vi "Meas Result Update View.vi"(8 "error in":errorcluster, 10 "gui refs":T29, 11 "meas":T3={"swp cfg"={"N"=0, "R"=0, "f list"=[], "smpl delay"=0.0, "set delay"=0.0, "set delay np"=0.0, "meas root"=path "", "meas name"="", "meas a-index"=FALSE, "rnd sweep"=FALSE, "mode"=enum."Frequency", "swp mode"=enum."Linear", "avg"=0, "subrec"=0, "multi-freq"=FALSE, "selfcal"=FALSE, "selfcal period [h]"=0.0}, "bridge"={"type"=enum."TWM client", "TWM"={"pipe name"="", "parameters"=[], "handle"=0, "fixed aper [s]"=0.0, "f-list [Hz]"=[], "discrete f-list"=FALSE, "unc mode"=enum."None", "unc mcc"=0, "unc first"=FALSE, "alg id"=enum."TWM-LowZ - Low Z measurement"}, "last f"=0.0, "bias comp"={"bias type"=enum."dummy", "VISA"="", "Enable"=FALSE, "channel qu"=[], "channel Uinit"=[]}, "sim mode"=enum."Generic RLC network", "channel idns"=[], "sim phases"=1}, "src"={"type"=enum."Tektronix AFG3101C", "afg"={"VISA"="", "const"=0.0, "gen DC"=FALSE, "ext ref"=FALSE}, "cDAQ dds"={"device"="", "channels"=[], "mclk source"="", "mclk [Hz]"=0.0, "fs [Hz]"=0.0, "block [s]"=0.0, "buf [s]"=0.0, "task"="", "cmd queue"=refnum, "proc ref"=refnum, "smpl clock out"="/cDAQ3/PFI0", "export smpl clock"=FALSE, "DC ofs [V]"=[], "timebase source"="", "timebase mode"=enum."Local", "dither"=enum."Disabled", "dither level"=0.0, "phase [rad]"=[]}, "gain [V/A]"=1.0, "F5xxx session"={"VISA"="", "mode"=enum."AC voltage", "Earth on"=FALSE, "Ext ref lock"=FALSE}}, "results"=refnum, "dvm"={"type"=enum."Disabled", "F5790"={"VISA"="", "Input"=enum."input 1", "Digital filter restart"=enum."medium", "hi resolution"=enum."off", "Digital filter mode"=enum."off", "ext guard"=FALSE}}} {"src"."cDAQ dds"."channels" min=0 step=1; "bridge"."TWM"."f-list [Hz]" format="%#_6p"; "swp cfg"."f list"."bias" format="%#_3p"; "swp cfg"."f list"."level" format="%#_3p"; "swp cfg"."f list"."fs [Hz]" format="%#_5p"; "swp cfg"."f list"."time [s]" format="%#_3p"; "swp cfg"."f list"."f/fs" format="%#_3p"; "swp cfg"."f list"."periods" format="%#_3f"; "swp cfg"."f list"."f [Hz]" format="%#_5p"}) -> (0 "error out":errorcluster, 3 "was modified?":bool)   [LabVIEW 2020]
doc: "Update results view."
uses:
  Meas Result GUI References.ctl
  Meas Result Freq Format.ctl
  Meas Results Sweep Data Uncertainty Mode.ctl
  Meas Result 4TP Impedance Mode.ctl
  Impedance Equivalent Circuit.ctl
  meas session.ctl
  Meas Sweep Config.ctl
  Meas Freq Info.ctl
  meas_swp_mode.ctl
  meas_sweep_flist_mode.ctl
  bridge/Bridge Session.ctl
  bridge/Bridge Type.ctl
  drivers/TWM client/TWM Session.ctl
  drivers/TWM client/TWM parameters.ctl
  drivers/TWM client/Meas Proc QWTB Uncertainty Mode.ctl
  bridge/Bridge Algorithm.ctl
  bridge/Bridge Bias Session.ctl
  bridge/Bridge Bias Type.ctl
  bridge/Bridge Sim Mode.ctl
  source/Source Session.ctl
  source/Source Type.ctl
  drivers/AFG3101C/AFG3101C Session.ctl
  drivers/cDAQ DDS/cDAQ DDS Session.ctl
  drivers/cDAQ DDS/cDAQ DDS Setup.ctl
  drivers/cDAQ DDS/cDAQ DDS Timebase Mode.ctl
  drivers/cDAQ DDS/cDAQ DDS Dither.ctl
  drivers/Fluke 5XXX/top_lev/F5xxx_session.ctl
  drivers/Fluke 5XXX/top_lev/F5xxx_output_mode.ctl
  Meas Results Ref.ctl
  Meas Results.ctl
  bridge/Bridge Frequency Readings Data.ctl
  drivers/TWM client/Meas Proc QWTB Spectrum Data.ctl
  drivers/TWM client/TWM Phase Info.ctl
  dvm/dvm session.ctl
  dvm/dvm type.ctl
  drivers/Fluke 5790A/top_level/F5790 session.ctl
  Meas Result Major Format.ctl
  Meas Result Deviation Format.ctl
  varilib/varilib.lvlib
panel:
  in  "mjr dev fmt":T1 caption="Enum"
  in  "mjr fmt":T2=enum."%_5p"
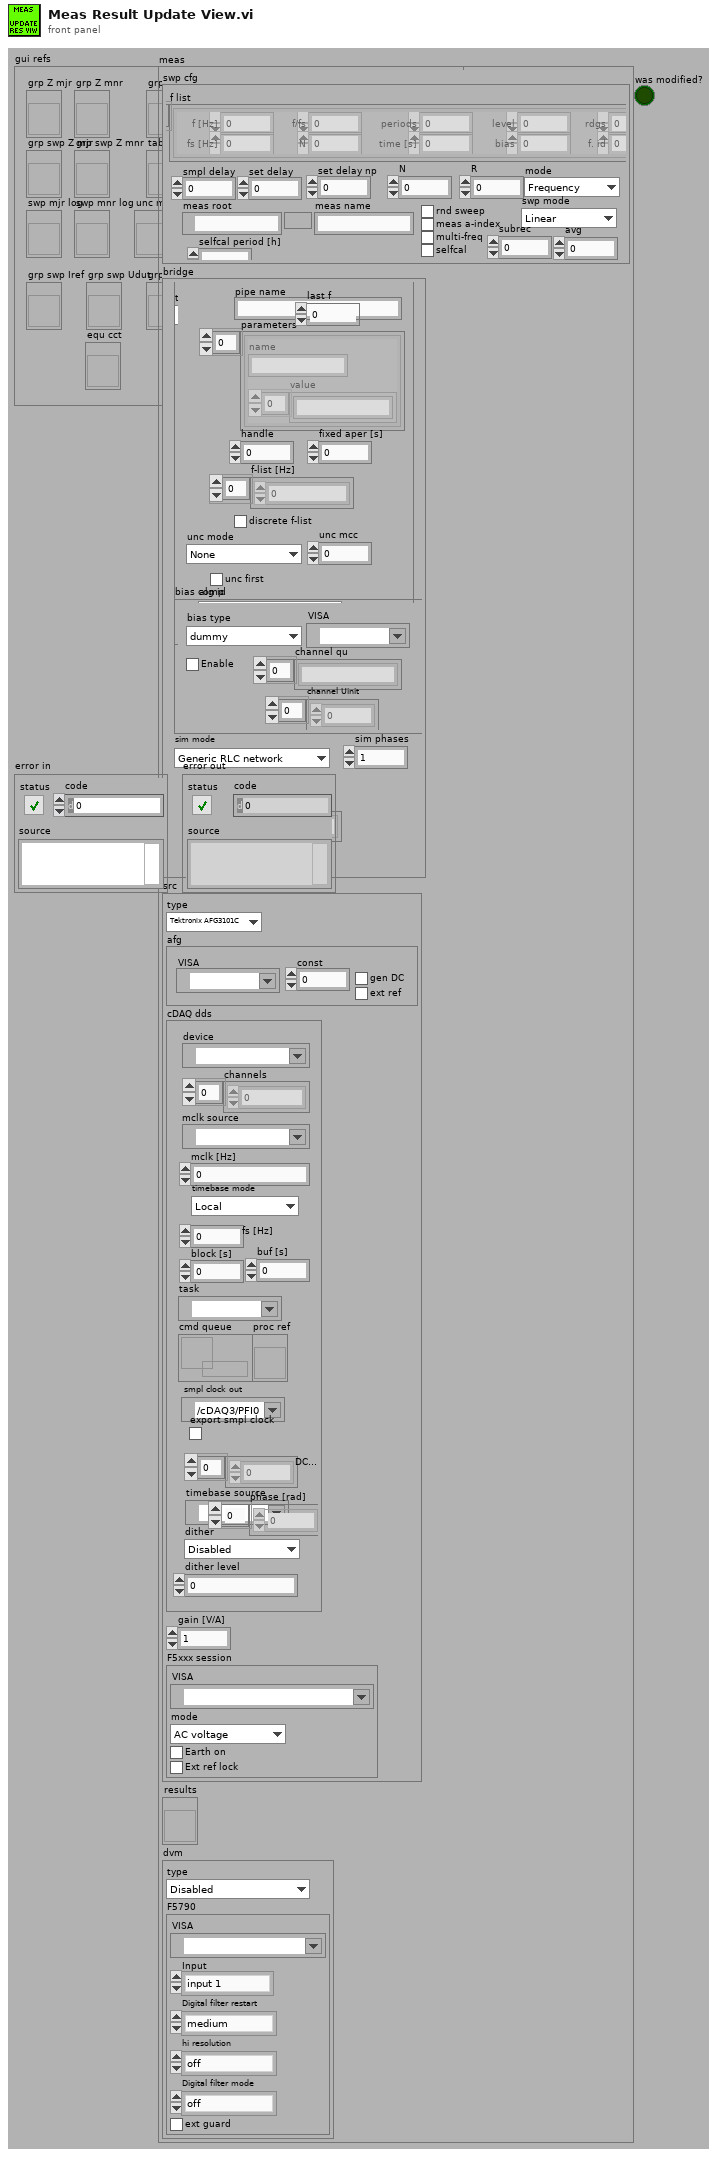
[diagram p1: front panel]
types:
  T1 = typedef "Meas Result Deviation Format.ctl" = enum16{"dev(abs)", "dev(%)", "dev(ppm)", "u(abs)", "u(%)", "u(ppm)"}
  T2 = typedef "Meas Result Major Format.ctl" = enum16{"%_3p", "%_4p", "%_5p", "%_6p", "%_7p", "%_8p", "%_5f", "%_6f", "%_7f", "%_8f", "%_5e", "%_6e", "%_7e", "%_8e", "%.4f", "%.5f", "%.6f", "%.7f"}
  T3 = typedef "meas session.ctl" = cluster{"swp cfg":T4, "bridge":T8, "src":T17, "results":T25, "dvm":T26}
  T4 = typedef "Meas Sweep Config.ctl" = cluster{"N":i32, "R":i32, "f list":T5[], "smpl delay":dbl, "set delay":dbl, "set delay np":dbl, "meas root":path, "meas name":string, "meas a-index":bool, "rnd sweep":bool, "mode":T6, "swp mode":T7, "avg":i32, "subrec":i32, "multi-freq":bool, "selfcal":bool, "selfcal period [h]":dbl}
  T5 = typedef "Meas Freq Info.ctl" = cluster{"f [Hz]":dbl, "periods":dbl, "f/fs":dbl, "time [s]":dbl, "fs [Hz]":dbl, "N":i32, "level":dbl, "bias":dbl, "rdgs":i32, "f. id":i32}
  T6 = typedef "meas_swp_mode.ctl" = enum16{"Frequency", "Level", "Bias"}
  T7 = typedef "meas_sweep_flist_mode.ctl" = enum16{"Linear", "Log10"}
  T8 = typedef "Bridge Session.ctl" = cluster{"type":T9, "TWM":T10, "last f":dbl, "bias comp":T14, "sim mode":T16, "channel idns":string[], "sim phases":i32}
  T9 = typedef "Bridge Type.ctl" = enum16{"TWM client", "dummy"}
  T10 = typedef "TWM Session.ctl" = cluster{"pipe name":string, "parameters":T11[], "handle":i32, "fixed aper [s]":dbl, "f-list [Hz]":dbl[], "discrete f-list":bool, "unc mode":T12, "unc mcc":i32, "unc first":bool, "alg id":T13}
  T11 = typedef "TWM parameters.ctl" = cluster{"name":string, "value":string[]}
  T12 = typedef "Meas Proc QWTB Uncertainty Mode.ctl" = enum16{"None", "GUF", "Monte Carlo"}
  T13 = typedef "Bridge Algorithm.ctl" = enum16{"TWM-LowZ - Low Z measurement", "TWM-InpZ - Digitizer input Z measurement", "TWM-TIAZ - High Z using TIA"}
  T14 = typedef "Bridge Bias Session.ctl" = cluster{"bias type":T15, "VISA":refnum<visa-resource-name>, "Enable":bool, "channel qu":string[], "channel Uinit":dbl[]}
  T15 = typedef "Bridge Bias Type.ctl" = enum16{"dummy", "CMI LiBbias V1.0"}
  T16 = typedef "Bridge Sim Mode.ctl" = enum16{"Generic RLC network", "Interchannel transfer", "Input impedance"}
  T17 = typedef "Source Session.ctl" = cluster{"type":T18, "afg":T19, "cDAQ dds":T20, "gain [V/A]":dbl, "F5xxx session":T23}
  T18 = typedef "Source Type.ctl" = enum16{"Tektronix AFG3101C", "cDAQ DAC", "Fluke 5xxx", "Agilent 33120A", "dummy"}
  T19 = typedef "AFG3101C Session.ctl" = cluster{"VISA":refnum<visa-resource-name>, "const":dbl, "gen DC":bool, "ext ref":bool}
  T20 = typedef "cDAQ DDS Session.ctl" = cluster{"device":tag, "channels":i32[], "mclk source":tag, "mclk [Hz]":dbl, "fs [Hz]":dbl, "block [s]":dbl, "buf [s]":dbl, "task":refnum<k21>, "cmd queue":refnum<queue>, "proc ref":refnum<vi>, "smpl clock out":tag, "export smpl clock":bool, "DC ofs [V]":dbl[], "timebase source":tag, "timebase mode":T21, "dither":T22, "dither level":dbl, "phase [rad]":dbl[]}
  T21 = typedef "cDAQ DDS Timebase Mode.ctl" = enum16{"Local", "Take from ADC (e.g. NI 9238)", "Other source"}
  T22 = typedef "cDAQ DDS Dither.ctl" = enum16{"Disabled", "Gaussian"}
  T23 = typedef "F5xxx_session.ctl" = cluster{"VISA":refnum<visa-resource-name>, "mode":T24, "Earth on":bool, "Ext ref lock":bool}
  T24 = typedef "F5xxx_output_mode.ctl" = enum16{"AC voltage", "AC current"}
  T25 = typedef "Meas Results Ref.ctl" = refnum<vi>
  T26 = typedef "dvm session.ctl" = cluster{"type":T27, "F5790":T28}
  T27 = typedef "dvm type.ctl" = enum16{"Disabled", "Simulated", "Fluke 5790A"}
  T28 = typedef "F5790 session.ctl" = cluster{"VISA":refnum<visa-resource-name>, "Input":enum16{"input 1", "input 2", "wide-band"}, "Digital filter restart":enum16{"medium", "fine", "coarse"}, "hi resolution":enum16{"off", "on"}, "Digital filter mode":enum16{"off", "fast", "medium", "slow"}, "ext guard":bool}
  T29 = typedef "Meas Result GUI References.ctl" = cluster{"grp Z mjr":refnum<vi>, "grp Z mnr":refnum<vi>, "grp swp Z mjr":refnum<vi>, "grp swp Z mnr":refnum<vi>, "swp mjr log":refnum<vi>, "swp mnr log":refnum<vi>, "grp ref":refnum<vi>, "tab swp":refnum<vi>, "mjr fmt":refnum<vi>, "mnr fmt":refnum<vi>, "mjr dev fmt":refnum<vi>, "mnr dev fmt":refnum<vi>, "res frq fmt":refnum<vi>, "unc mode":refnum<vi>, "mode 4TP":refnum<vi>, "grp spec 0":refnum<vi>, "grp spec 1":refnum<vi>, "cb spec log":refnum<vi>, "res pid":refnum<vi>, "res fid":refnum<vi>, "grp swp cplx":refnum<vi>, "cb grp inv Xs":refnum<vi>, "grp swp Iref":refnum<vi>, "grp swp Udut":refnum<vi>, "grp swp Udvm":refnum<vi>, "swp Iref log":refnum<vi>, "swp Udut log":refnum<vi>, "swp Udvm log":refnum<vi>, "grp ui ref":refnum<vi>, "grp Iref":refnum<vi>, "grp Udut":refnum<vi>, "grp Udvm":refnum<vi>, "equ cct":refnum<vi>}
  T30 = typedef "Meas Results.ctl" = cluster{"freqs":T31[][], "locked":bool, "last fid":i32, "modified":bool, "mjr name":string, "mnr name":string, "last spectra":T32[][], "saved?":bool, "TWM phase":T33[], "time start":timestamp, "time stop":timestamp, "equ cct":string}
  T31 = typedef "Bridge Frequency Readings Data.ctl" = cluster{"Udut":dbl[], "Iref":dbl[], "Udc":dbl[], "Idc":dbl[], "mjr":dbl[], "mnr":dbl[], "mjr_sh":dbl[], "mnr_sh":dbl[], "u(mjr)":dbl[], "u(mnr)":dbl[], "ua2(mjr)":dbl[], "ua2(mnr)":dbl[], "n":i32, "f [Hz]":dbl, "fs [Hz]":dbl, "aperture [s]":dbl, "Udvm":dbl[], "u(Udvm) [V]":dbl}
  T32 = typedef "Meas Proc QWTB Spectrum Data.ctl" = cluster{"x":sgl[], "y":sgl[], "label":string}
  T33 = typedef "TWM Phase Info.ctl" = cluster{"ref chn id (I)":string, "dut chn id (U)":string, "ref chn range [V]":dbl, "dut chn range [V]":dbl, "aperture [s]":dbl, "fs [Hz]":dbl, "ref chn transducer (I)":string, "dut chn transducer (U)":string}
  T34 = typedef "Impedance Equivalent Circuit.ctl" = enum16{"Keep original", "Rs-Xs", "Gp-Bp", "Z-phid", "Z-phir", "Y-phid", "Y-phir", "Cp-D", "Cp-Q", "Cp-Rp", "Cp-Gp", "Cs-D", "Cs-Q", "Cs-Rs", "Ls-Rs", "Ls-Q", "Rs-Tau"}
  T35 = typedef "Meas Result 4TP Impedance Mode.ctl" = enum16{"4T/4TP total Z", "4TP-shield Z"}
  T36 = typedef "Impedance Equivalent Circuit Type Info.ctl" = cluster{"major":string, "major unit":string, "minor":string, "minor unit":string, "combined":string, "major+unit":string, "minor+unit":string}
  T37 = typedef "Meas Results Sweep Data Uncertainty Mode.ctl" = enum16{"ua(y)", "ua(y) (p=95%)", "uc(y) (p=95%)"}
  T38 = typedef "Meas Quantity Names.ctl" = cluster{"mjr name":string, "mnr name":string, "mjr unit":string, "mnr unit":string, "mjr full":string, "mnr full":string}
  T39 = typedef "Meas Results Sweep Data.ctl" = cluster{"Udut":dbl[], "Iref":dbl[], "Udc":dbl[], "Idc":dbl[], "mjr":dbl[], "mnr":dbl[], "mjr_sh":dbl[], "mnr_sh":dbl[], "f [Hz]":dbl[], "n [-]":i32[], "fs [Hz]":dbl[], "aperture [s]":dbl[], "Udvm":dbl[]}
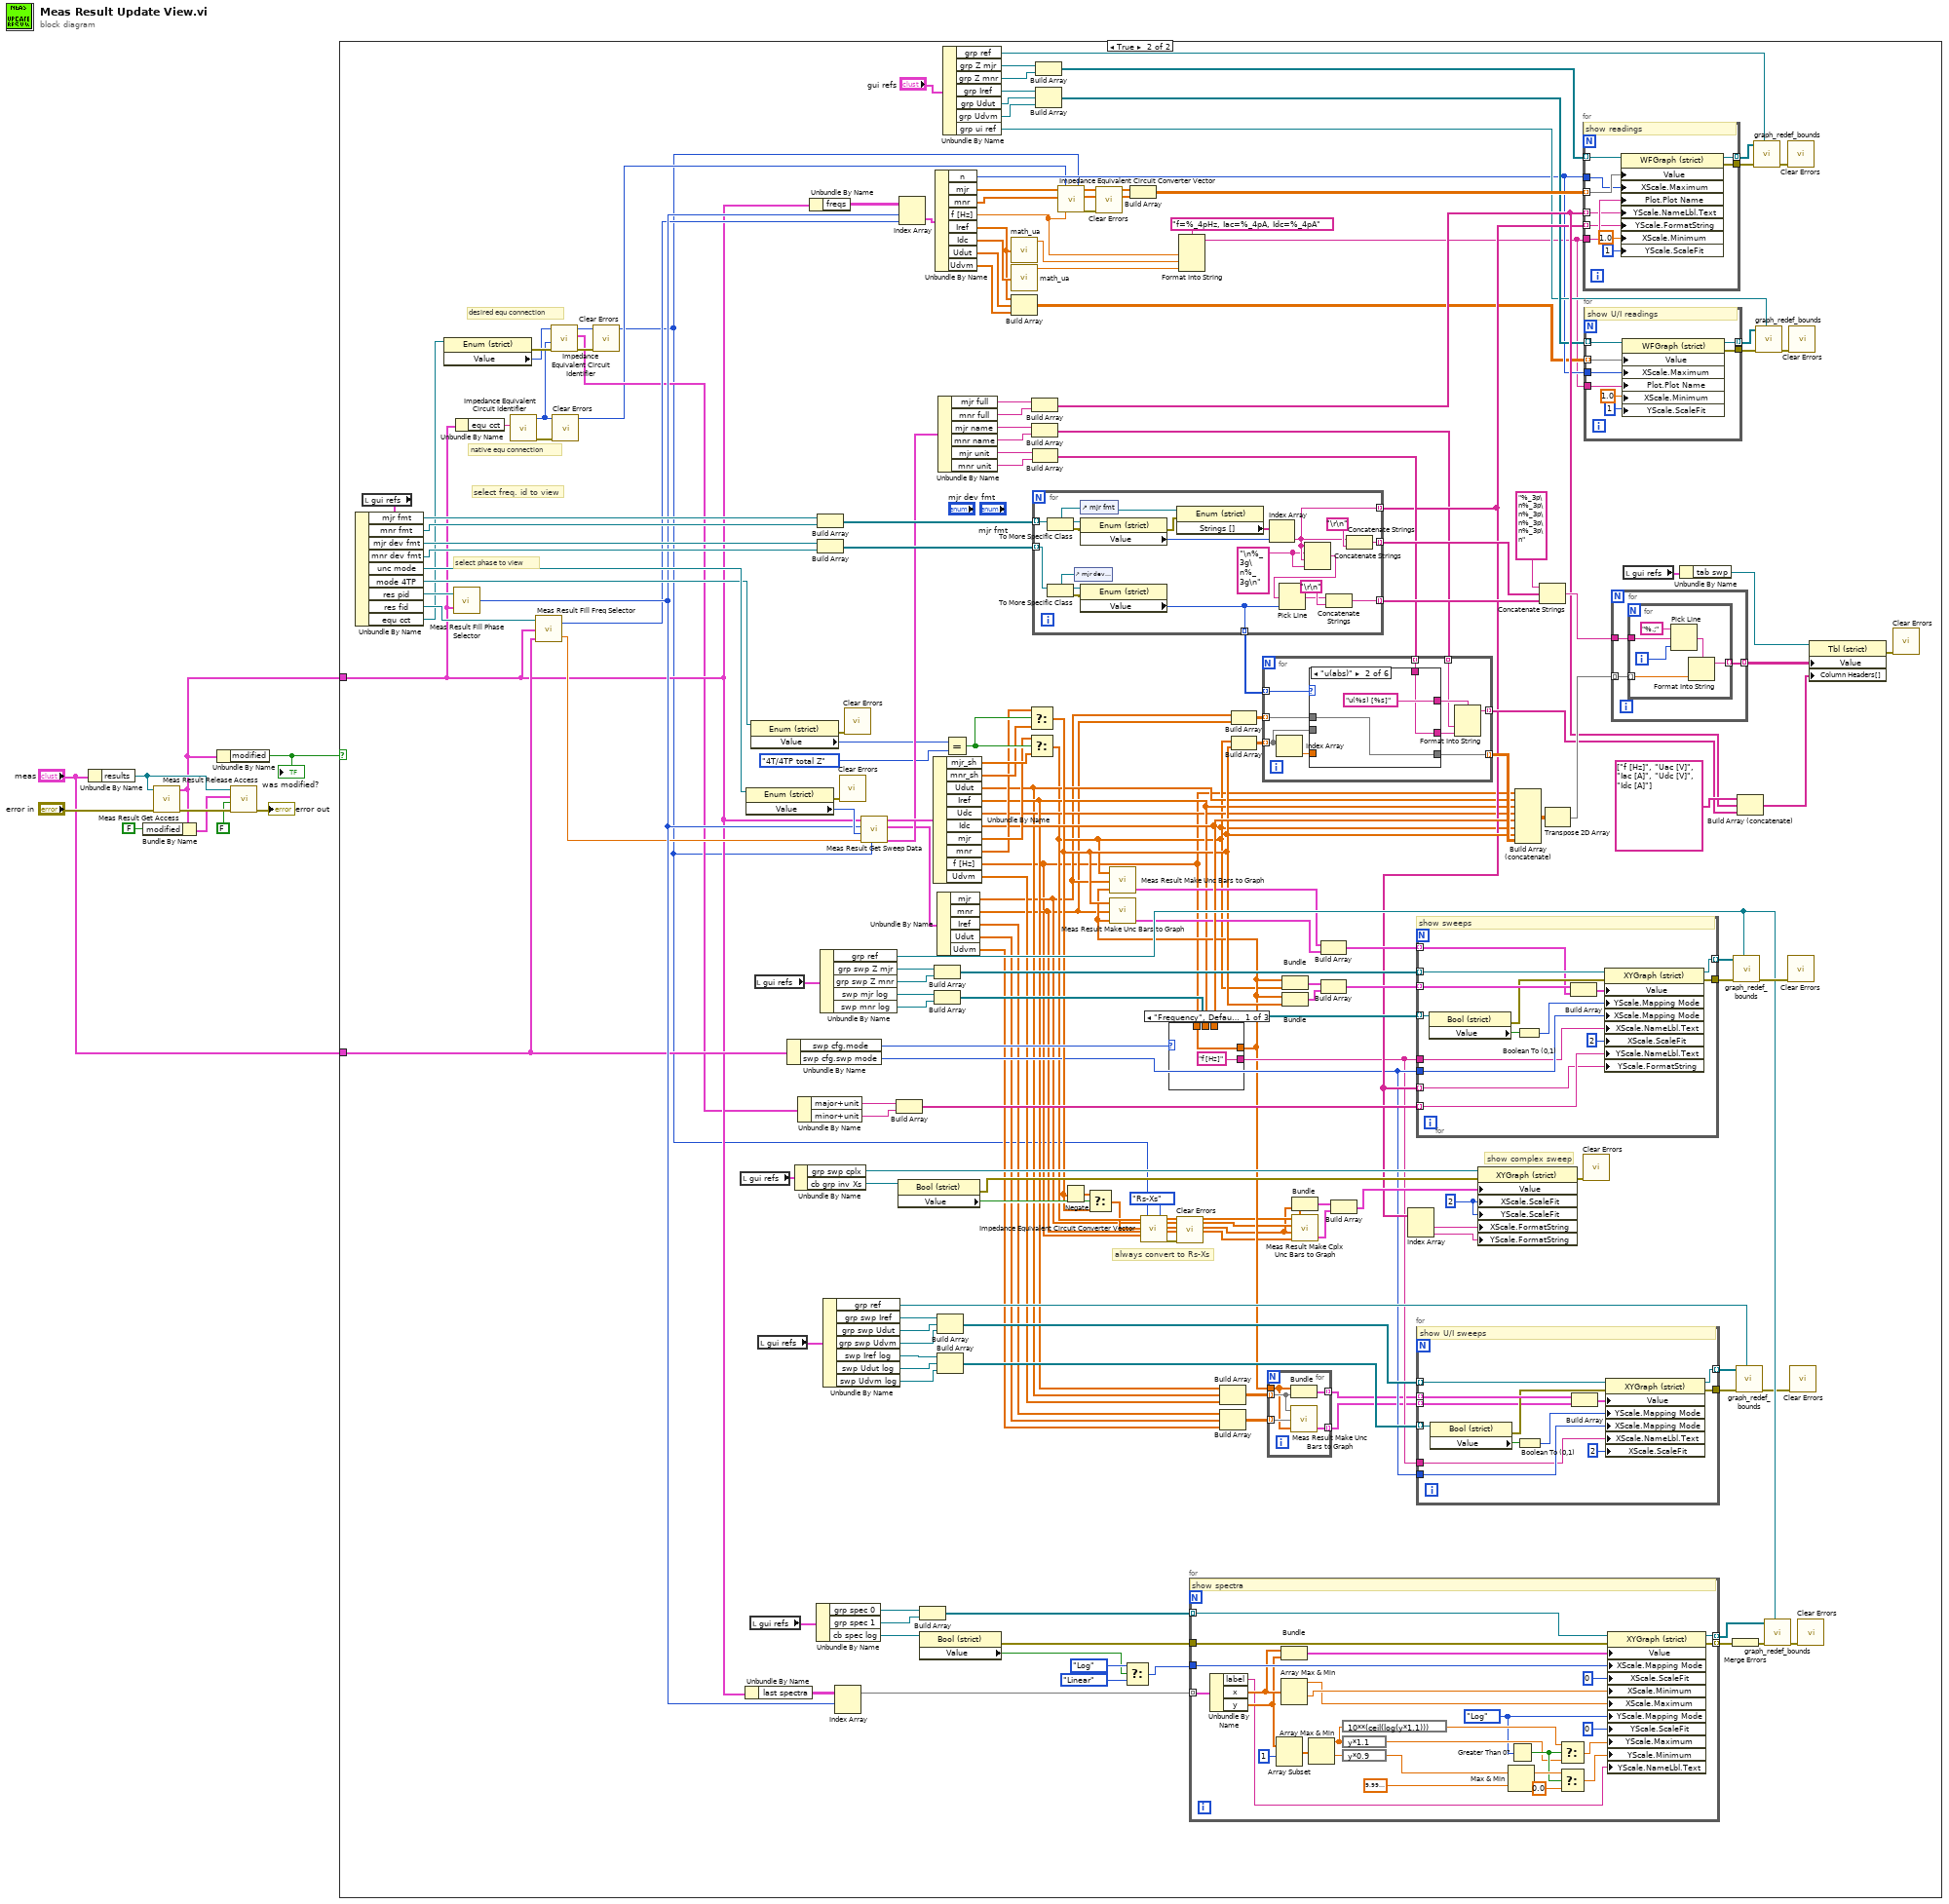
[diagram p0: block diagram]
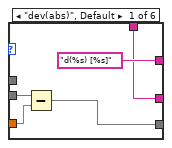
[diagram p3: hidden frame]
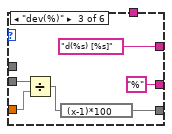
[diagram p4: hidden frame]
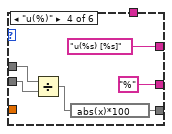
[diagram p5: hidden frame]
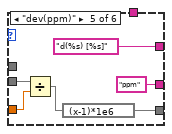
[diagram p6: hidden frame]
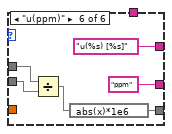
[diagram p7: hidden frame]
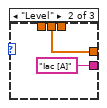
[diagram p8: hidden frame]
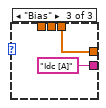
[diagram p9: hidden frame]
diagram:
  n1 = Unbundle By Name("meas") -> ("results"=w9:T25)
  n2 = call "Meas Result Get Access.vi"("error in"="error in", "results ref"=w9) -> ("error out"=w10:errorcluster, "results data"=w2:T30)  [unwired: 8 in]
  n3 = Bundle By Name(cluster=w2, "modified"=FALSE) -> (w5:T30)
  n4 = Unbundle By Name(w2) -> ("modified"=w6:bool)
  "was modified?" <- w6
  n5 = call "Meas Result Release Access.vi"("error in"=w10, "Release only (True)"=FALSE, "results data in"=w5, "results ref"=w9) -> ("error out"=→"error out":errorcluster)  [unwired: 7 in]
  n6 = case shown="True" w6 {
    tunnel: w2 -> [_ w31]
    tunnel: "meas" -> [_ w99]
    frame False {
    }
    frame True {
      w83 = u8 2 ("X Scale.Scale Fit")
      # "always convert to Rs-Xs"
      # "desired equ connection"
      # "native equ connection"
      # "show complex sweep"
      # "select freq. id to view"
      # "select phase to view"
      n7 = local read "gui refs"() -> (w164:T29)
      n8 = Unbundle By Name(w164) -> ("mjr fmt"=w163:refnum<vi>, "mnr fmt"=w162:refnum<vi>, "mjr dev fmt"=w160:refnum<vi>, "mnr dev fmt"=w159:refnum<vi>, "unc mode"=w146:refnum<vi>, "mode 4TP"=w131:refnum<vi>, "res pid"=w105:refnum<vi>, "res fid"=w102:refnum<vi>, "equ cct"=w37:refnum<vi>)
      n9 = property class="Enum (strict)"(reference=w37) -> (error out=w29:errorcluster, "Value"=w28:T34)  [unwired: 1 in, 1 out]
      n10 = call "Meas Result Fill Phase Selector.vi"("results data"=w31, "res pid"=w105) -> ("phase index (default: 0)"=w103:u16)
      n11 = Unbundle By Name(w31) -> ("equ cct"=w30:string)
      n12 = call "Impedance Equivalent Circuit Identifier.vi"("type in by string"=w30) -> ("error out"=w32:errorcluster, "type out"=w13:T34)  [unwired: 8 in, 1 out]
      n13 = call "Meas Result Fill Freq Selector.vi"("meas"=w99, "results data"=w31, "res fid"=w102) -> ("freq filter (NaN: no filter)"=w100:dbl, "freq index (default: 0)"=w101:u16)
      n14 = call "Impedance Equivalent Circuit Identifier.vi"("error in (no error)"=w29, "type in original"=w13, "type in"=w28) -> ("error out"=w27:errorcluster, "type info"=w26:T36, "type out"=w12:T34)  [unwired: 6 in]
      n15 = call <vilib>:"Clear Errors.vi"("error in (no error)"=w32) -> ()  [unwired: 5 in, 2 out]
      n16 = call <vilib>:"Clear Errors.vi"("error in (no error)"=w27) -> ()  [unwired: 5 in, 2 out]
      n17 = local read "gui refs"() -> (w95:T29)
      n18 = Unbundle By Name(w31) -> ("last spectra"=w116:T32[][])
      n19 = property class="Enum (strict)"(reference=w146) -> (error out=w144:errorcluster, "Value"=w145:T37)  [unwired: 1 in, 1 out]
      n20 = local read "gui refs"() -> (w122:T29)
      n21 = property class="Enum (strict)"(reference=w131) -> (error out=w130:errorcluster, "Value"=w129:T35)  [unwired: 1 in, 1 out]
      n22 = local read "gui refs"() -> (w193:T29)
      n23 = local read "gui refs"() -> (w72:T29)
      n24 = Unbundle By Name(w99) -> ("swp cfg.mode"=w186:T6, "swp cfg.swp mode"=w66:T7)
      n25 = Unbundle By Name(w95) -> ("grp swp cplx"=w93:refnum<vi>, "cb grp inv Xs"=w94:refnum<vi>)
      n26 = Unbundle By Name(w26) -> ("major+unit"=w147:string, "minor+unit"=w148:string)
      n27 = Unbundle By Name(w31) -> ("freqs"=w199:T31[][])
      n28 = Unbundle By Name(w122) -> ("grp spec 0"=w121:refnum<vi>, "grp spec 1"=w120:refnum<vi>, "cb spec log"=w119:refnum<vi>)
      n29 = Build Array(w163, w162) -> (w161:refnum<vi>[])
      n30 = Build Array(w160, w159) -> (w158:refnum<vi>[])
      n31 = Unbundle By Name(w193) -> ("grp ref"=w111:refnum<vi>, "grp swp Z mjr"=w192:refnum<vi>, "grp swp Z mnr"=w191:refnum<vi>, "swp mjr log"=w185:refnum<vi>, "swp mnr log"=w184:refnum<vi>)
      n32 = Unbundle By Name(w72) -> ("grp ref"=w71:refnum<vi>, "grp swp Iref"=w73:refnum<vi>, "grp swp Udut"=w74:refnum<vi>, "grp swp Udvm"=w70:refnum<vi>, "swp Iref log"=w75:refnum<vi>, "swp Udut log"=w76:refnum<vi>, "swp Udvm log"=w69:refnum<vi>)
      n33 = Index Array(array=w116, index (row)=w103) -> (element=w104:T32[])  [unwired: 1 in]
      n34 = call <vilib>:"Clear Errors.vi"("error in (no error)"=w144) -> ()  [unwired: 5 in, 2 out]
      n35 = call <vilib>:"Clear Errors.vi"("error in (no error)"=w130) -> ()  [unwired: 5 in, 2 out]
      n36 = call "Meas Result Get Sweep Data.vi"("equ connection override"=w12, "freq filter (NaN: no filter)"=w100, "uncertainty mode"=w145, "phase index (default: 0)"=w103, "result"=w31) -> ("quantities"=w141:T38, "unc(data)"=w38:T39, "data"=w165:T39)  [unwired: 4 in]
      n37 = Build Array(w147, w148) -> (w96:string[])
      n38 = property class="Bool (strict)"(reference=w94) -> (error out=w92:errorcluster, "Value"=w91:bool)  [unwired: 1 in, 1 out]
      n39 = Index Array(array=w199, index (row)=w103, index (col)=w101) -> (element=w195:T31)
      n40 = Build Array(w121, w120) -> (w117:refnum<vi>[])
      n41 = property class="Bool (strict)"(reference=w119) -> (error out=w118:errorcluster, "Value"=w108:bool)  [unwired: 1 in, 1 out]
      n42 = Unbundle By Name(w165) -> ("mjr_sh"=w127:dbl[], "mnr_sh"=w125:dbl[], "Udut"=w53:dbl[], "Iref"=w63:dbl[], "Udc"=w62:dbl[], "Idc"=w106:dbl[], "mjr"=w124:dbl[], "mnr"=w123:dbl[], "f [Hz]"=w21:dbl[], "Udvm"=w61:dbl[])
      n43 = Build Array(w192, w191) -> (w190:refnum<vi>[])
      n44 = Build Array(w185, w184) -> (w183:refnum<vi>[])
      n45 = Unbundle By Name(w195) -> ("n"=w41:i32, "mjr"=w36:dbl[], "mnr"=w35:dbl[], "f [Hz]"=w15:dbl, "Iref"=w49:dbl[], "Idc"=w167:dbl[], "Udut"=w48:dbl[], "Udvm"=w47:dbl[])
      n46 = Unbundle By Name(w38) -> ("mjr"=w23:dbl[], "mnr"=w22:dbl[], "Iref"=w59:dbl[], "Udut"=w58:dbl[], "Udvm"=w57:dbl[])
      n47 = Build Array(w73, w74, w70) -> (w68:refnum<vi>[])
      n48 = Build Array(w75, w76, w69) -> (w67:refnum<vi>[])
      n49 = Unbundle By Name(w141) -> ("mjr full"=w150:string, "mnr full"=w149:string, "mjr name"=w140:string, "mnr name"=w139:string, "mjr unit"=w138:string, "mnr unit"=w137:string)
      n50 = Unbundle By Name("gui refs") -> ("grp ref"=w176:refnum<vi>, "grp Z mjr"=w198:refnum<vi>, "grp Z mnr"=w197:refnum<vi>, "grp Iref"=w46:refnum<vi>, "grp Udut"=w45:refnum<vi>, "grp Udvm"=w44:refnum<vi>, "grp ui ref"=w42:refnum<vi>)
      n51 = Equal?(x=w129, y=Meas_Result_4TP_Impedance_Mode."4T/4TP total Z") -> (x = y?=w126:bool)
      n52 = call "math_ua.vi"("x"=w49) -> ("mean(x)"=w166:dbl)  [unwired: 3 out]
      n53 = call "math_ua.vi"("x"=w167) -> ("mean(x)"=w168:dbl)  [unwired: 3 out]
      n54 = Build Array(w49, w48, w47) -> (w40:dbl[][])
      n55 = Select(t=w123, s=w126, f=w125) -> (s? t:f=w89:dbl[])
      n56 = Select(t=w124, s=w126, f=w127) -> (s? t:f=w25:dbl[])
      n57 = Build Array(w150, w149) -> (w134:string[])
      n58 = Build Array(w140, w139) -> (w80:string[])
      n59 = Build Array(w138, w137) -> (w136:string[])
      n60 = for {
        tunnel: w161 -> [w316] mode=indexing
        tunnel: [w305] -> w157 mode=indexing
        tunnel: w158 -> [w308] mode=indexing
        tunnel: [w300] -> w154 mode=indexing
        tunnel: [w299] -> w152 mode=indexing
        tunnel: [w298] -> w84 mode=indexing
        w297 = "\n%_3g\n%_3g\n"
        n61 = control-ref of="mjr dev fmt"() -> (w306:refnum<vi>)
        n62 = To More Specific Class(target class=w306, reference=w308) -> (specific class reference=w309:refnum<vi>, error out=w310:errorcluster)  [unwired: 1 in]
        n63 = control-ref of="mjr fmt"() -> (w307:refnum<vi>)
        n64 = To More Specific Class(target class=w307, reference=w316) -> (specific class reference=w315:refnum<vi>, error out=w314:errorcluster)  [unwired: 1 in]
        n65 = property class="Enum (strict)"(reference=w315, error in=w314) -> (error out=w311:errorcluster, "Value"=w312:T2)  [unwired: 1 out]
        n66 = property class="Enum (strict)"(reference=w309, error in=w310) -> ("Value"=w299:T1)  [unwired: 2 out]
        n67 = property class="Enum (strict)"(reference=w307, error in=w311) -> ("Strings []"=w313:string[])  [unwired: 2 out]
        n68 = Index Array(array=w313, index=w312) -> (element=w298:string)
        n69 = Concatenate Strings(w298, w297, w298, w297) -> (w302:string)
        n70 = Pick Line(multi-line string=w302, line index=w299) -> (output string=w301:string)  [unwired: 1 in]
        n71 = Concatenate Strings(w301, "\r\n") -> (w300:string)
        n72 = Concatenate Strings(w298, "\r\n") -> (w305:string)
      }
      n73 = Build Array(w198, w197) -> (w196:refnum<vi>[])
      n74 = Build Array(w46, w45, w44) -> (w43:refnum<vi>[])
      n75 = call "Impedance Equivalent Circuit Converter Vector.vi"("major in"=w36, "minor in"=w35, "type in"=w13, "f scalar [Hz]"=w15, "type out"=w12) -> ("major out"=w34:dbl[], "minor out"=w33:dbl[], "error out"=w16:errorcluster)  [unwired: 9 in, 3 out]
      n76 = Negate(x=w89) -> (-x=w90:dbl[])
      n77 = Select(t=w90, s=w91, f=w89) -> (s? t:f=w24:dbl[])
      n78 = call <vilib>:"Clear Errors.vi"("error in (no error)"=w16) -> ()  [unwired: 5 in, 2 out]
      n79 = Select(t=enum16{"Linear", "Log"}."Log" ("xlog"), s=w108, f=enum16{"Linear", "Log"}."Linear" ("xlog")) -> (s? t:f=w107:enum16{"Linear", "Log"})
      n80 = Build Array(w34, w33) -> (w194:dbl[][])
      n81 = call "Impedance Equivalent Circuit Converter Vector.vi"("major in"=w25, "u(major) in"=w23, "minor in"=w24, "u(minor) in"=w22, "f [Hz]"=w21, "type in"=w12, "type out"=Impedance_Equivalent_Circuit."Rs-Xs") -> ("major out"=w18:dbl[], "u(major) out"=w19:dbl[], "minor out"=w17:dbl[], "u(minor) out"=w20:dbl[], "error out"=w14:errorcluster)  [unwired: 7 in, 1 out]
      n82 = case shown="\"Frequency\", Default" w186 {
        tunnel: [w327 w329 w331] -> w64
        tunnel: w21 -> [w327 _ _]
        tunnel: w63 -> [_ w329 _]
        tunnel: w106 -> [_ _ w331]
        tunnel: ["f [Hz]" "Iac [A]" "Idc [A]"] -> w65
        frame "Frequency", Default {
        }
        frame "Level" {
        }
        frame "Bias" {
        }
      }
      n83 = call "Meas Result Make Unc Bars to Graph.vi"("independent"=w64, "unc"=w23, "mean"=w25) -> ("trace"=w98:cluster{dbl[], dbl[]})  [unwired: 2 out]
      n84 = call "Meas Result Make Unc Bars to Graph.vi"("independent"=w64, "unc"=w22, "mean"=w89) -> ("trace"=w97:cluster{dbl[], dbl[]})  [unwired: 2 out]
      n85 = call <vilib>:"Clear Errors.vi"("error in (no error)"=w14) -> ()  [unwired: 5 in, 2 out]
      n86 = Format Into String(format string="f=%_4pHz, Iac=%_4pA, Idc=%_4pA", w15, w166, w168) -> (resulting string=w39:string)  [unwired: 2 in, 1 out]
      n87 = for {
        tunnel: w118 -> [w254]
        tunnel: w104 -> [w248] mode=indexing
        tunnel: w117 -> [w253] mode=indexing
        tunnel: w107 -> [w252]
        tunnel: [w250] -> w113 mode=indexing
        tunnel: [w249] -> w112 mode=indexing
        w227 = enum16{"Linear", "Log"}."Log" ("xlog")
        # "show spectra"
        n88 = Unbundle By Name(w248) -> ("label"=w233:string, "x"=w236:sgl[], "y"=w235:sgl[])
        n89 = Array Subset(array=w235, index=1) -> (w244:sgl[])  [unwired: 1 in]
        n90 = Bundle("x"=w236, "y"=w235) -> (w234:cluster{"x":sgl[], "y":sgl[]})  [unwired: 1 in]
        n91 = Array Max & Min(array=w236) -> (max value=w246:sgl, min value=w247:sgl)  [unwired: 2 out]
        n92 = Array Max & Min(array=w244) -> (max value=w230:sgl, min value=w242:sgl)  [unwired: 2 out]
        n93 = expression code="10**(ceil(log(y*1.1)))"(w230) -> (w229:sgl)
        n94 = expression code="y*1.1"(w230) -> (w231:sgl)
        n95 = expression code="y*0.9"(w242) -> (w241:sgl)
        n96 = Max & Min(x=w241, y=sgl 1e-08) -> (max(x,y)=w239:sgl)  [unwired: 1 out]
        n97 = Greater Than 0?(x=w227) -> (x > 0?=w232:bool)
        n98 = Select(t=w229, s=w232, f=w231) -> (s? t:f=w228:sgl)
        n99 = Select(t=w239, s=w232, f=sgl 0.0) -> (s? t:f=w238:sgl)
        n100 = property class="XYGraph (strict)"(reference=w253, error in=w254, "Value"=w234, "XScale.Mapping Mode"=w252, "XScale.ScaleFit"=u8 0 ("X Scale.Scale Fit"), "XScale.Minimum"=w247, "XScale.Maximum"=w246, "YScale.Mapping Mode"=w227, "YScale.ScaleFit"=u8 0 ("Y Scale.Scale Fit"), "YScale.Maximum"=w228, "YScale.Minimum"=w238, "YScale.NameLbl.Text"=w233) -> (reference out=w249:refnum<vi>, error out=w250:errorcluster)
      }
      n101 = Build Array(w63, w53, w61) -> (w60:dbl[][])
      n102 = Build Array(w59, w58, w57) -> (w56:dbl[][])
      n103 = Build Array(w23, w22) -> (w142:dbl[][])
      n104 = Build Array(w25, w89) -> (w153:dbl[][])
      n105 = for {
        tunnel: w153 -> [w260] mode=indexing
        tunnel: w152 -> [w264] mode=indexing
        tunnel: [w262] -> w151 mode=indexing
        tunnel: w142 -> [w261] mode=indexing
        tunnel: [w258] -> w133 mode=indexing
        tunnel: w80 -> [w257] mode=indexing
        tunnel: w136 -> [w255] mode=indexing
        n106 = Index Array(array=w260) -> (element=w263:dbl)  [unwired: 1 in]
        n107 = case shown="\"u(abs)\"" w264 {
          tunnel: w263 -> [w269 _ w277 _ w289 _]
          tunnel: [w268 w272 w276 w283 w288 w295] -> w262
          tunnel: w261 -> [_ w272 _ w282 _ w294]
          tunnel: w260 -> [w267 _ w275 w281 w287 w293]
          tunnel: ["d(%s) [%s]" "u(%s) [%s]" "d(%s) [%s]" "u(%s) [%s]" "d(%s) [%s]" "u(%s) [%s]"] -> w259
          tunnel: [w265 w270 "%" ("mnr unit") "%" ("mnr unit") "ppm" ("mnr unit") "ppm" ("mnr unit")] -> w256
          tunnel: w255 -> [w265 w270 _ _ _ _]
          frame "dev(abs)", Default {
            n108 = Subtract(x=w267, y=w269) -> (x-y=w268:dbl[])
          }
          frame "u(abs)" {
          }
          frame "dev(%)" {
            n109 = Divide(x=w275, y=w277) -> (x/y=w278:dbl[])
            n110 = expression code="(x-1)*100"(w278) -> (w276:dbl[])
          }
          frame "u(%)" {
            n111 = Divide(x=w282, y=w281) -> (x/y=w284:dbl[])
            n112 = expression code="abs(x)*100"(w284) -> (w283:dbl[])
          }
          frame "dev(ppm)" {
            n113 = Divide(x=w287, y=w289) -> (x/y=w290:dbl[])
            n114 = expression code="(x-1)*1e6"(w290) -> (w288:dbl[])
          }
          frame "u(ppm)" {
            n115 = Divide(x=w294, y=w293) -> (x/y=w296:dbl[])
            n116 = expression code="abs(x)*1e6"(w296) -> (w295:dbl[])
          }
        }
        n117 = Format Into String(format string=w259, w257, w256) -> (resulting string=w258:string)  [unwired: 2 in, 1 out]
      }
      n118 = for {
        tunnel: w64 -> [w211]
        tunnel: w60 -> [w213] mode=indexing
        tunnel: w56 -> [w212] mode=indexing
        tunnel: [w210] -> w54 mode=indexing
        tunnel: [w209] -> w55 mode=indexing
        n119 = Bundle("Idc"=w211, w213) -> (w209:cluster{"Idc":dbl[], dbl[]})  [unwired: 1 in]
        n120 = call "Meas Result Make Unc Bars to Graph.vi"("independent"=w211, "unc"=w212, "mean"=w213) -> ("trace"=w210:cluster{dbl[], dbl[]})  [unwired: 2 out]
      }
      n121 = Bundle("Idc"=w64, "mjr_sh"=w25) -> (w189:cluster{"Idc":dbl[], "mjr_sh":dbl[]})  [unwired: 1 in]
      n122 = Bundle("Idc"=w64, "mnr_sh"=w89) -> (w188:cluster{"Idc":dbl[], "mnr_sh":dbl[]})  [unwired: 1 in]
      n123 = Bundle("major out"=w18, "minor out"=w17) -> (w88:cluster{"major out":dbl[], "minor out":dbl[]})  [unwired: 1 in]
      n124 = call "Meas Result Make Cplx Unc Bars to Graph.vi"("unc y"=w20, "y"=w17, "unc x"=w19, "x"=w18) -> ("trace"=w86:cluster{dbl[], dbl[]})  [unwired: 2 out]
      n125 = Build Array(w98, w97) -> (w143:cluster{dbl[], dbl[]}[])
      n126 = Build Array(w189, w188) -> (w187:cluster{"Idc":dbl[], "mnr_sh":dbl[]}[])
      n127 = Build Array(w88, w86) -> (w87:cluster{"major out":dbl[], "minor out":dbl[]}[])
      n128 = Index Array(array=w84) -> (element #1=w82:string, element #2=w81:string)  [unwired: 2 in]
      n129 = for {
        tunnel: w190 -> [w346] mode=indexing
        tunnel: w187 -> [w344] mode=indexing
        tunnel: w183 -> [w343] mode=indexing
        tunnel: w66 -> [w339]
        tunnel: [w338] -> w179
        tunnel: [w337] -> w178 mode=indexing
        tunnel: w65 -> [w336]
        tunnel: w96 -> [w334] mode=indexing
        tunnel: w143 -> [w333] mode=indexing
        tunnel: w84 -> [w332] mode=indexing
        # "show sweeps"
        n130 = property class="Bool (strict)"(reference=w343) -> (error out=w342:errorcluster, "Value"=w341:bool)  [unwired: 1 in, 1 out]
        n131 = Boolean To (0,1)(Boolean=w341) -> (0, 1=w340:i16)
        n132 = Build Array(w344, w333) -> (w345:cluster{"Idc":dbl[], "mnr_sh":dbl[]}[])
        n133 = property class="XYGraph (strict)"(reference=w346, error in=w342, "Value"=w345, "YScale.Mapping Mode"=w340, "XScale.Mapping Mode"=w339, "XScale.NameLbl.Text"=w336, "XScale.ScaleFit"=u8 2 ("X Scale.Scale Fit"), "YScale.NameLbl.Text"=w334, "YScale.FormatString"=w332) -> (reference out=w337:refnum<vi>, error out=w338:errorcluster)
      }
      n134 = for {
        tunnel: w68 -> [w226] mode=indexing
        tunnel: w55 -> [w224] mode=indexing
        tunnel: w67 -> [w223] mode=indexing
        tunnel: w66 -> [w219]
        tunnel: [w218] -> w77
        tunnel: [w217] -> w78 mode=indexing
        tunnel: w65 -> [w216]
        tunnel: w54 -> [w214] mode=indexing
        # "show U/I sweeps"
        n135 = property class="Bool (strict)"(reference=w223) -> (error out=w222:errorcluster, "Value"=w221:bool)  [unwired: 1 in, 1 out]
        n136 = Boolean To (0,1)(Boolean=w221) -> (0, 1=w220:i16)
        n137 = Build Array(w224, w214) -> (w225:cluster{"Idc":dbl[], dbl[]}[])
        n138 = property class="XYGraph (strict)"(reference=w226, error in=w222, "Value"=w225, "YScale.Mapping Mode"=w220, "XScale.Mapping Mode"=w219, "XScale.NameLbl.Text"=w216, "XScale.ScaleFit"=u8 2 ("X Scale.Scale Fit")) -> (reference out=w217:refnum<vi>, error out=w218:errorcluster)
      }
      n139 = property class="XYGraph (strict)"(reference=w93, error in=w92, "Value"=w87, "XScale.ScaleFit"=w83, "YScale.ScaleFit"=w83, "XScale.FormatString"=w82, "YScale.FormatString"=w81) -> (error out=w85:errorcluster)  [unwired: 1 out]
      n140 = Build Array (concatenate)(w21, w53, w63, w62, w106, w25, w89, w151) -> (w175:dbl[][])
      n141 = Concatenate Strings("%_3p\n%_3p\n%_3p\n%_3p\n%_3p\n", w157, w154) -> (w155:string)
      n142 = Transpose 2D Array(2D array=w175) -> (transposed array=w174:dbl[][])
      n143 = for {
        tunnel: w196 -> [w356] mode=indexing
        tunnel: w194 -> [w355] mode=indexing
        tunnel: [w354] -> w182
        tunnel: [w353] -> w180 mode=indexing
        tunnel: w41 -> [w352]
        tunnel: w39 -> [w351]
        tunnel: w134 -> [w350] mode=indexing
        tunnel: w84 -> [w349] mode=indexing
        # "show readings"
        n144 = property class="WFGraph (strict)"(reference=w356, "Value"=w355, "XScale.Maximum"=w352, "Plot.Plot Name"=w351, "YScale.NameLbl.Text"=w350, "YScale.FormatString"=w349, "XScale.Minimum"=1.0 ("X Scale.Range:Minimum"), "YScale.ScaleFit"=u8 1 ("X Scale.Scale Fit")) -> (reference out=w353:refnum<vi>, error out=w354:errorcluster)  [unwired: 1 in]
      }
      n145 = call <vilib>:"Clear Errors.vi"("error in (no error)"=w85) -> ()  [unwired: 5 in, 2 out]
      n146 = for {
        tunnel: w43 -> [w208] mode=indexing
        tunnel: w40 -> [w207] mode=indexing
        tunnel: [w206] -> w50
        tunnel: [w205] -> w52 mode=indexing
        tunnel: w41 -> [w204]
        tunnel: w39 -> [w203]
        # "show U/I readings"
        n147 = property class="WFGraph (strict)"(reference=w208, "Value"=w207, "XScale.Maximum"=w204, "Plot.Plot Name"=w203, "XScale.Minimum"=1.0 ("X Scale.Range:Minimum"), "YScale.ScaleFit"=u8 1 ("X Scale.Scale Fit")) -> (reference out=w205:refnum<vi>, error out=w206:errorcluster)  [unwired: 1 in]
      }
      n148 = for {
        tunnel: w155 -> [w319]
        tunnel: w174 -> [w318] mode=indexing
        tunnel: [w317] -> w171 mode=indexing
        n149 = for {
          tunnel: w319 -> [w325]
          tunnel: [w322] -> w317 mode=indexing
          tunnel: w318 -> [w321] mode=indexing
          i -> [w320]
          n150 = Pick Line(string ("")="%.;", multi-line string=w325, line index=w320) -> (output string=w324:string)
          n151 = Format Into String(format string=w324, w321) -> (resulting string=w322:string)  [unwired: 2 in, 1 out]
        }
      }
      n152 = local read "gui refs"() -> (w173:T29)
      n153 = Unbundle By Name(w173) -> ("tab swp"=w172:refnum<vi>)
      n154 = Merge Errors(w113) -> (w114:errorcluster)
      n155 = call "graph_redef_bounds.vi"("grp ref pos"=w111, "error in"=w179, "graph refs in"=w178) -> ("error out"=w177:errorcluster)  [unwired: 7 in, 1 out]
      n156 = call "graph_redef_bounds.vi"("grp ref pos"=w71, "error in"=w77, "graph refs in"=w78) -> ("error out"=w79:errorcluster)  [unwired: 7 in, 1 out]
      n157 = Build Array (concatenate)(string[] ["f [Hz]", "Uac [V]", "Iac [A]", "Udc [V]", "Idc [A]"], w134, w133) -> (w132:string[])
      n158 = call "graph_redef_bounds.vi"("grp ref pos"=w176, "error in"=w182, "graph refs in"=w180) -> ("error out"=w181:errorcluster)  [unwired: 7 in, 1 out]
      n159 = call "graph_redef_bounds.vi"("grp ref pos"=w42, "error in"=w50, "graph refs in"=w52) -> ("error out"=w51:errorcluster)  [unwired: 7 in, 1 out]
      n160 = call "graph_redef_bounds.vi"("grp ref pos"=w111, "error in"=w114, "graph refs in"=w112) -> ("error out"=w115:errorcluster)  [unwired: 7 in, 1 out]
      n161 = call <vilib>:"Clear Errors.vi"("error in (no error)"=w181) -> ()  [unwired: 5 in, 2 out]
      n162 = call <vilib>:"Clear Errors.vi"("error in (no error)"=w177) -> ()  [unwired: 5 in, 2 out]
      n163 = call <vilib>:"Clear Errors.vi"("error in (no error)"=w51) -> ()  [unwired: 5 in, 2 out]
      n164 = call <vilib>:"Clear Errors.vi"("error in (no error)"=w79) -> ()  [unwired: 5 in, 2 out]
      n165 = call <vilib>:"Clear Errors.vi"("error in (no error)"=w115) -> ()  [unwired: 5 in, 2 out]
      n166 = property class="Tbl (strict)"(reference=w172, "Value"=w171, "Column Headers[]"=w132) -> (error out=w170:errorcluster)  [unwired: 1 in, 1 out]
      n167 = call <vilib>:"Clear Errors.vi"("error in (no error)"=w170) -> ()  [unwired: 5 in, 2 out]
    }
  }
